vi "Make TTB.vi"(3 "Header file data":T1 {"Pixel depth" items=["8 bits", "16 bits", "Float", "Complex", "RGB", "HSL"]; "time of 1st frame, \nsec since 1/1/04" format="%.2f"}, 4 "error in (no error)":errorcluster, 5 "first frame number":u32, 6 "# of frames":u32, 7 "refnum":refnum<file>) -> (0 "error out":errorcluster)   [LabVIEW 2016]
doc: "Make TTB.vi\n\nThis VI takes an array of U32 integers (millisecond time stamps) and a double integer (time, in seconds, of the first frame, in regards to 1/1/04) and converts this information to a time table readable format and saves it to a time table."
uses:
  Header file data.ctl
  Seq file v 1/Offset table.ctl
  Seq file v 1/Offset.ctl
  Seq file v 1/file number.ctl
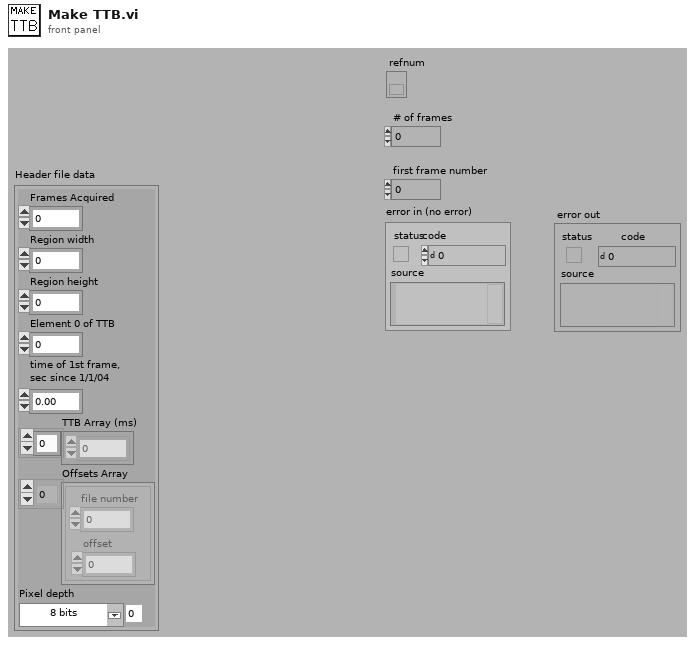
[diagram p1: front panel]
types:
  T1 = typedef "Header file data.ctl" = cluster{"Frames Acquired":u32, "Region width":i32, "Region height":i32, "Element 0 of TTB":u32, "time of 1st frame, \nsec since 1/1/04":dbl, "TTB Array (ms)":u32[], "Offsets Array":T2, "Pixel depth":u32}
  T2 = typedef "Offset table.ctl" = cluster{"offset":T3, "file number":T4}[]
  T3 = typedef "Offset.ctl" = i32
  T4 = typedef "file number.ctl" = u8
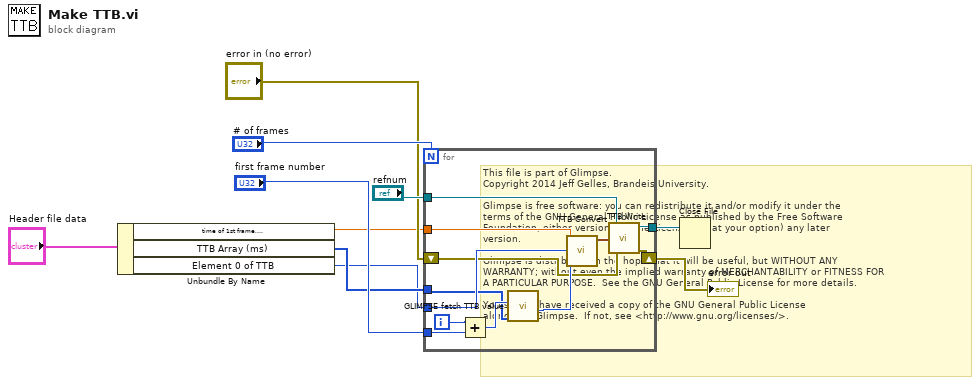
[diagram p0: block diagram]
diagram:
  # "This file is part of Glimpse. \nCopyright 2014 Jeff Gelles, Brandeis University.    \n\nGlimpse is free software: you can redistribute it and/or modify it under the \nterms of the GNU General Public License as published by the Free Software \nFoundation, either version 3 of the License, or (at your option) any later \nversion.\n\nGlimpse is distributed in the hope that it will be useful, but WITHOUT ANY \nWARRANTY; without even the implied warranty of MERCHANTABILITY or FITNESS FOR \nA PARTICULAR PURPOSE.  See the GNU General Public License for more details.\n\nYou should have received a copy of the GNU General Public License\nalong with Glimpse.  If not, see <http://www.gnu.org/licenses/>."
  n1 = Unbundle By Name("Header file data") -> ("time of 1st frame, \nsec since 1/1/04"=w4:dbl, "TTB Array (ms)"=w3:u32[], "Element 0 of TTB"=w2:u32)
  n2 = for {
    N: "# of frames" -> [_]
    tunnel: "refnum" -> [w22]
    tunnel: [w21] -> w10
    tunnel: w4 -> [w20]
    tunnel: w3 -> [w11]
    tunnel: w2 -> [w18]
    tunnel: "first frame number" -> [w15]
    shift-right: [w13] -> w6
    shift-left: "error in (no error)" -> [w14]
    i -> [w16]
    n3 = Add(x=w16, y=w15) -> (x+y=w12:u32)
    n4 = call "GLIMPSE fetch TTB value.vi"("Array of TTB Values (ms)"=w11, "Logical Frame Number\n(starting with zero)"=w12) -> ("TTB value out"=w17:u32)  [unwired: 6 out]
    n5 = call "TTB Convert.vi"("time of 1st frame, sec since 1/1/04"=w20, "First element of TTB values"=w18, "Current element of TTB values"=w17) -> ("TTB Cluster Out"=w19:cluster{i32, u16, i16, i16})  [unwired: 5 out]
    n6 = call "TTB Write.vi"("error in"=w14, "TTB Cluster In"=w19, "refnum in"=w22) -> ("error out"=w13:errorcluster, "refnum out"=w21:refnum<file>)  [unwired: 3 out]
  }
  "error out" <- w6
  n7 = Close File(refnum=w10) -> ()  [unwired: 1 in, 2 out]
